vi "UnloadClassQueue.vi"(8 "ErrorIn(No Error)":errorcluster caption="entrée d'erreur (pas d'erreur)", 11 "BaseDevice.lvclass":refnum<class "BaseDevice.lvclass">) -> (0 "sortie d'erreur":errorcluster, 3 "BaseDevice.lvclass Out":refnum<class "BaseDevice.lvclass">)   [LabVIEW 2019, in "BaseDevice.lvclass"]
uses:
  BaseDevice.lvclass
  BaseDevice.lvclass/BaseDevice.ctl
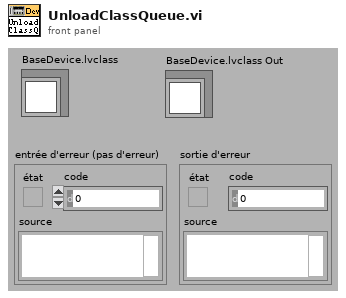
[diagram p1: front panel]
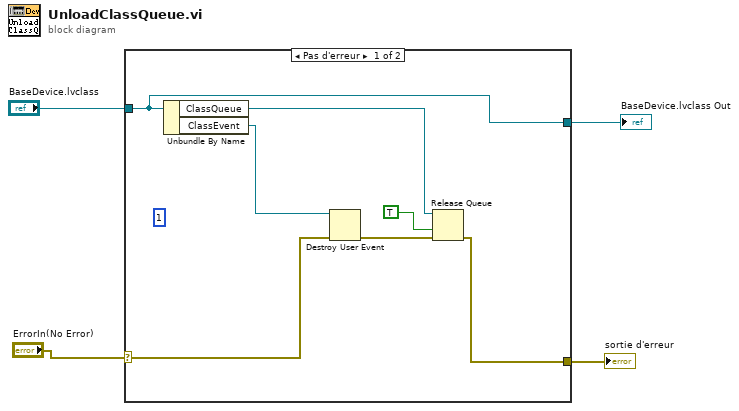
[diagram p0: block diagram]
diagram:
  n1 = case shown="Pas d'erreur" "ErrorIn(No Error)" {
    selector: "ErrorIn(No Error)" -> [w6 w13]
    tunnel: [w10 w13] -> w4
    tunnel: "BaseDevice.lvclass" -> [w9 w12]
    tunnel: [w9 w12] -> w1
    frame No Error {
      (unwired) 1 ("taille max de la file d'attente (-1, non limitée)")
      n2 = Unbundle By Name(w9) -> ("ClassQueue"=w11:refnum<queue>, "ClassEvent"=w8:refnum<user-event>)
      n3 = Destroy User Event(user event=w8, error in=w6) -> (error out=w7:errorcluster)
      n4 = Release Queue(queue=w11, force destroy? (F)=TRUE ("forcer la destruction ? (F)"), error in (no error)=w7) -> (error out=w10:errorcluster)  [unwired: 2 out]
    }
    frame Error {
    }
  }
  "sortie d'erreur" <- w4
  "BaseDevice.lvclass Out" <- w1
